vi "Cal image analysis prototype.vi"() -> ()   [LabVIEW 2017]
uses:
  <vilib>/Utility/miscctls.llb/LVPointTypeDef.ctl
  <vilib>/vision/NI_Vision_Development_Module.lvlib
panel:
  in  "Calculate":bool
  out "Index":i32
  in  "Index":i32(slide) scale=0.0..40.0
  out "MAX STD":T1(plugin-control)
  in  "Done":bool
  out "Array 1":T2(array[cluster])
  out "Mean values":sgl[](array[numeric]) format="%.2f"
  out "Standard deviations":sgl[](array[numeric]) format="%.2f"
  out "Array 2":T3(array[cluster])
  in  "Select Z-stack dataset folder":path=path "J:/UCL/Rig 3 MovCor integration version/Datasets/Z-stacks for AOL cal image analysis/Z-stacks for AOL cal image analysis-set 1/Zstack 1024-235-20um range-Laser 25 percent"
  # "Finds the sharpest image by looking at standard deviation.\nIt works well since the sharper/more focused the image the brighter it is."
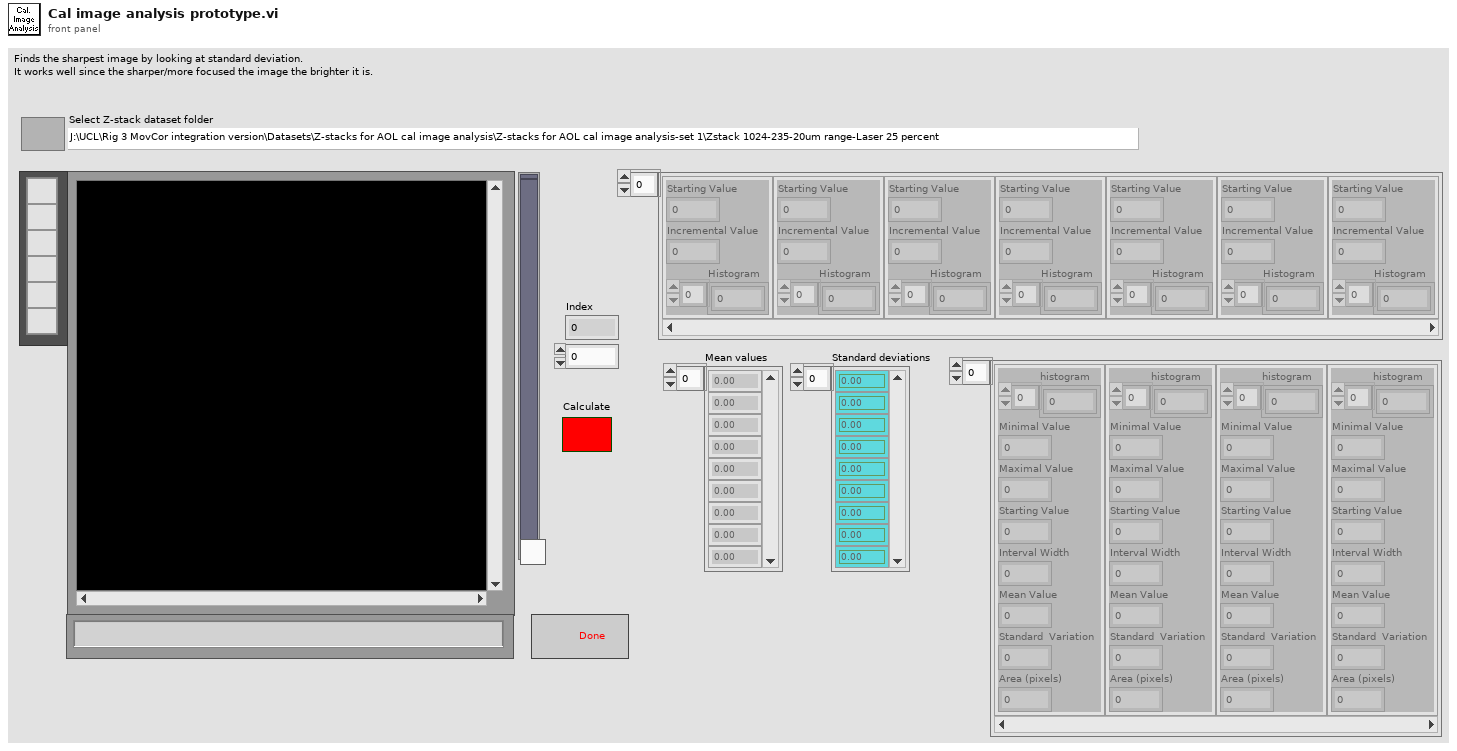
[diagram p1: front panel]
types:
  T1 = typedef "IMAQ Image.ctl" = refnum<image>
  T2 = cluster{"Starting Value":sgl, "Incremental Value":sgl, "Histogram":u32[]}[]
  T3 = cluster{"histogram":u32[], "Minimal Value":sgl, "Maximal Value":sgl, "Starting Value":sgl, "Interval Width":sgl, "Mean Value":sgl, "Standard  Variation":sgl, "Area (pixels)":i32}[]
  T4 = typedef "LVPointTypeDef.ctl" = cluster{"Horizontal":i16, "Vertical":i16}
  T5 = cluster{"Starting Value":sgl, "Incremental Value":sgl, "Histogram":u32[]}
  T6 = cluster{"histogram":u32[], "Minimal Value":sgl, "Maximal Value":sgl, "Starting Value":sgl, "Interval Width":sgl, "Mean Value":sgl, "Standard  Variation":sgl, "Area (pixels)":i32}
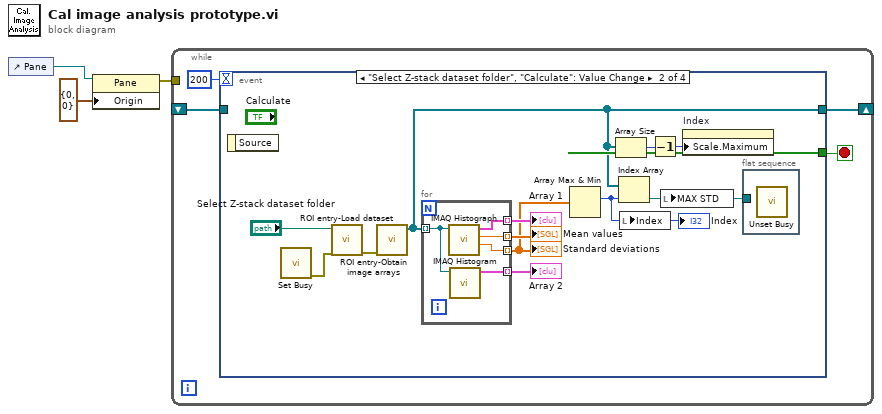
[diagram p0: block diagram]
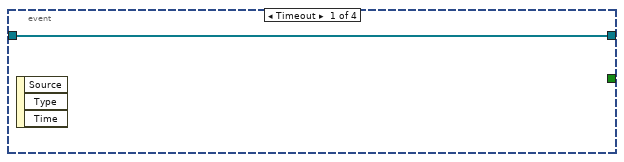
[diagram p2: hidden frame]
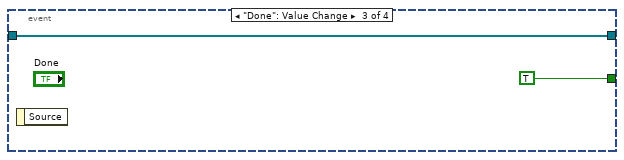
[diagram p3: hidden frame]
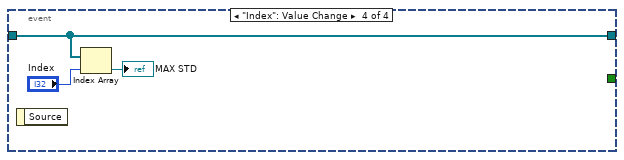
[diagram p4: hidden frame]
diagram:
  n1 = control-ref of="Pane"() -> (w2:refnum<vi>)
  n2 = property class="Pane"(reference=w2, "Origin"=T4 {"Horizontal"=0, "Vertical"=0}) -> (error out=w1:errorcluster)  [unwired: 1 in, 1 out]
  n3 = while {
    tunnel: w1 -> [_]
    shift-right: [w5] -> _
    shift-left: _ -> [w4]
    stop <- w7 stop-if-true
    n4 = event shown="[1] \"Select Z-stack dataset folder\", \"Calculate\": Value Change" {
      selector: _ -> [_ _ _ _]
      dyn-events: _ -> [_ _ _ _]
      timeout: 200 -> [_ _ _ _]
      tunnel: [_ _ TRUE ("Done") _] -> w7
      tunnel: [w8 w9 w26 w29] -> w5
      tunnel: w4 -> [w8 _ w26 w29]
      event Timeout {
        n5 = event-data() -> ()  [unwired: 1 in, 3 out]
      }
      event "Select Z-stack dataset folder", "Calculate": Value Change {
        n6 = event-data() -> ()  [unwired: 1 in, 1 out]
        n7 = call <vilib>:"Set Busy.vi"() -> ("error out"=w12:errorcluster)  [unwired: 10 in, 1 out]
        n8 = call "ROI entry-Load dataset.vi"("error in (no error)"=w12, "Experiment folder path OR Z-stack folder path"="Select Z-stack dataset folder") -> ("error out"=w13:errorcluster)  [unwired: 9 in]
        n9 = call "ROI entry-Obtain image arrays.vi"("error in (no error)"=w13) -> ("RedImageArray"=w9:T1[])  [unwired: 9 in, 1 out]
        n10 = for {
          tunnel: w9 -> [w25] mode=indexing
          tunnel: [w24] -> w17 mode=indexing
          tunnel: [w23] -> w16 mode=indexing
          tunnel: [w22] -> w10 mode=indexing
          tunnel: [w21] -> w15 mode=indexing
          n11 = call "IMAQ Histograph"("Image"=w25) -> ("Standard  Deviation"=w22:sgl, "Mean Value"=w23:sgl, "Histogram Graph"=w24:T5)  [unwired: 7 in, 1 out]
          n12 = call "IMAQ Histogram"("Image"=w25) -> ("Histogram Report"=w21:T6)  [unwired: 9 in, 1 out]
        }
        "Array 2" <- w15
        "Standard deviations" <- w10
        "Mean values" <- w16
        "Array 1" <- w17
        n13 = Array Max & Min(array=w10) -> (max index (indices)=w18:i32)  [unwired: 3 out]
        "Index" <- w18
        n14 = Array Size(array=w9) -> (size(s)=w19:i32)
        n15 = Index Array(array=w9, index=w18) -> (element=w11:T1)
        n16 = local write "Index"(w18) -> ()
        n17 = Decrement(x=w19) -> (x-1=w20:i32)
        n18 = local write "MAX STD"(w11) -> ()
        n19 = property on="Index" class="Slide (strict)"("Scale.Maximum"=w20) -> ()  [unwired: 2 in, 2 out]
        n20 = flat-sequence {
          tunnel: w11 -> [_]
          frame #0 {
            n21 = call <vilib>:"Unset Busy.vi"() -> ()  [unwired: 11 in, 1 out]
          }
        }
      }
      event "Done": Value Change {
        n22 = event-data() -> ()  [unwired: 1 in, 1 out]
      }
      event "Index": Value Change {
        n23 = event-data() -> ()  [unwired: 1 in, 1 out]
        n24 = Index Array(array=w29, index="Index") -> (element=→"MAX STD":T1)
      }
    }
  }
